vi "Write Parts.vi"(8 "error in (no error)":errorcluster, 10 "Parts":T1[](array[typedef]), 11 "Multipart Upload in":refnum<class "Multipart Upload.lvclass">) -> (0 "error out":errorcluster, 3 "Multipart Upload out":refnum<class "Multipart Upload.lvclass">)   [LabVIEW 2015, in "NI_AWS_S3.lvlib" / "Multipart Upload.lvclass"]
uses:
  Multipart Upload.lvclass
  Part.ctl
  Multipart Upload.lvclass/Multipart Upload.ctl
  NI_AWS_S3.lvlib
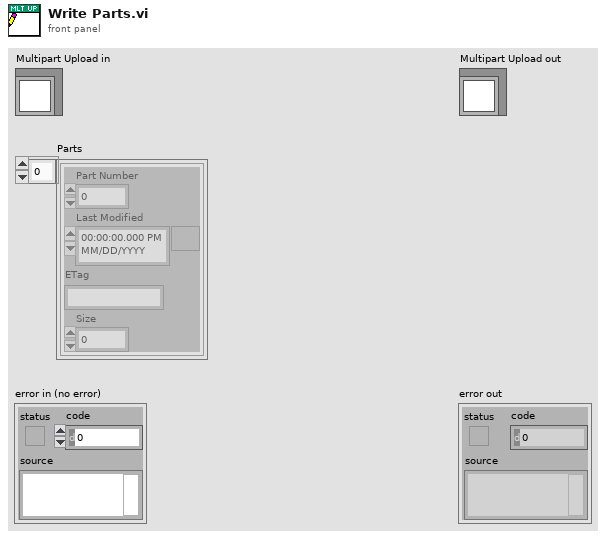
[diagram p1: front panel]
types:
  T1 = typedef "NI_AWS_S3.lvlib/Part.ctl" = cluster{"Part Number":i32, "Last Modified":timestamp, "ETag":string, "Size":u64}
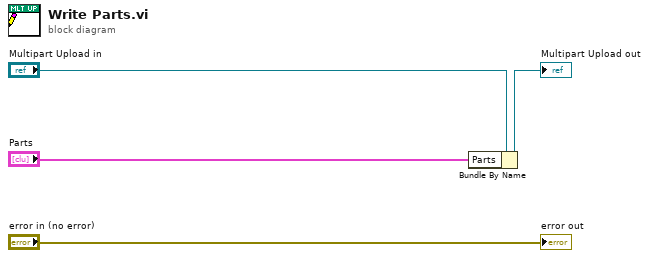
[diagram p0: block diagram]
diagram:
  n1 = Bundle By Name(cluster="Multipart Upload in", "Parts"="Parts") -> (→"Multipart Upload out":refnum<class "Multipart Upload.lvclass">)
  "error out" <- "error in (no error)"
